vi "GV DO5.vi"() -> ()   [LabVIEW 2017]
panel:
  out "DO5":bool
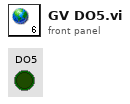
[diagram p1: front panel]
diagram:
